vi "getAllsubset.vi"(8 "error in (no error)":errorcluster, 10 "getAll":T1, 11 "instrument.PPMS-W-1 in":refnum<class "instrument.PPMS-W-1.lvclass">) -> (0 "error out":errorcluster, 2 "output cluster":variant, 3 "instrument.PPMS-W-1 out":refnum<class "instrument.PPMS-W-1.lvclass">)   [LabVIEW 2019, in "instrument.PPMS-W-1.lvclass"]
uses:
  instrument.PPMS-W-1.lvclass
  instrument.PPMS/Typedefs/PPMS.getAll--cluster.ctl
  instrument.PPMS/instrument.PPMS.lvclass
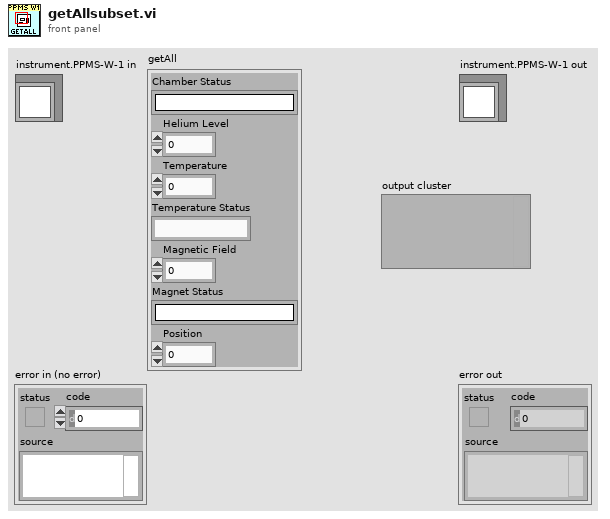
[diagram p1: front panel]
types:
  T1 = typedef "instrument.PPMS.lvclass/PPMS.getAll--cluster.ctl" = cluster{"Chamber Status":string, "Helium Level":dbl, "Temperature":dbl, "Temperature Status":string, "Magnetic Field":dbl, "Magnet Status":string, "Position":dbl}
  T2 = cluster{"Chamber Status":string, "Temperature":dbl, "Temperature Status":string, "Magnetic Field":dbl, "Magnet Status":string}
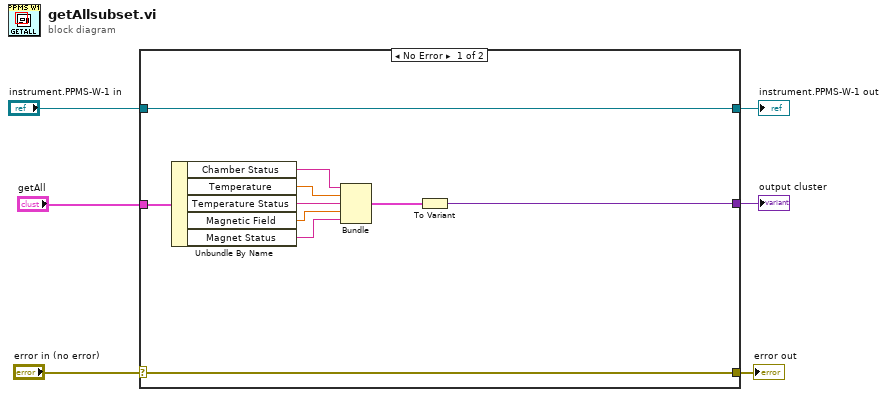
[diagram p0: block diagram]
diagram:
  n1 = case shown="No Error" "error in (no error)" {
    selector: "error in (no error)" -> [w15 w18]
    tunnel: [w15 w18] -> w6
    tunnel: [w16 w17] -> w4
    tunnel: "instrument.PPMS-W-1 in" -> [w16 w17]
    tunnel: "getAll" -> [w9 _]
    tunnel: [w14 _] -> w5
    frame No Error {
      n2 = Unbundle By Name(w9) -> ("Chamber Status"=w10:string, "Temperature"=w13:dbl, "Temperature Status"=w7:string, "Magnetic Field"=w12:dbl, "Magnet Status"=w11:string)
      n3 = Bundle("Chamber Status"=w10, "Temperature"=w13, "Temperature Status"=w7, "Magnetic Field"=w12, "Magnet Status"=w11) -> (w8:T2)  [unwired: 1 in]
      n4 = To Variant(anything=w8) -> (Variant=w14:variant)
    }
    frame Error {
    }
  }
  "error out" <- w6
  "instrument.PPMS-W-1 out" <- w4
  "output cluster" <- w5
